vi "UpdateTileSlide.vi"(8 "error in (no error)":errorcluster, 11 "Game in":refnum<class "Game.lvclass">) -> (0 "error out":errorcluster, 3 "Game out":refnum<class "Game.lvclass">)   [LabVIEW 2019, in "RT_Game.lvlib" / "Game.lvclass"]
uses:
  Game.lvclass
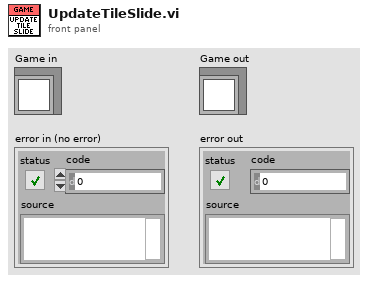
[diagram p1: front panel]
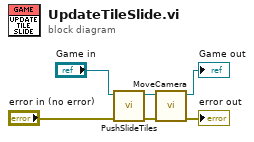
[diagram p0: block diagram]
diagram:
  n1 = call "PushSlideTiles.vi"("error in (no error)"="error in (no error)", "Game in"="Game in") -> ("error out"=w2:errorcluster, "Game out"=w1:refnum<class "Game.lvclass">)  [unwired: 8 in]
  n2 = call "MoveCamera.vi"("error in (no error)"=w2, "Game in"=w1) -> ("error out"=→"error out":errorcluster, "Game out"=→"Game out":refnum<class "Game.lvclass">)  [unwired: 8 in]
